vi "NI-DCPower Source DC Voltage T14.vi"() -> ()   [LabVIEW 2021, in "NI-DCPower Source DC Voltage T14.lvlib"]
doc: "Demonstrates how to use the DC Voltage Output Function to force an output voltage. This example initializes a session, configures the Output Function, Sense, Autorange, Voltage Level and Current Limit, initiates generation, waits for a specified delay, and measures the voltage and current output. This example uses Single Point source mode."
uses:
  NI-DCPower Source DC Voltage T14.lvlib
  <instrlib>/niDCPower/nidcpower.llb/niDCPower Source Mode.ctl
  <instrlib>/niDCPower/nidcpower.llb/niDCPower Wait For Event - Event.ctl
  <instrlib>/niDCPower/nidcpower.llb/niDCPower Output Function.ctl
panel:
  in  "error in":errorcluster
  out "error out":errorcluster
  in  "Source Delay (Sec)":dbl=0.1 format="%.3p"
  out "Voltage Measurement":dbl
  out "Current Measurement":dbl
  in  "Current Limit Range":dbl=0.01 format="%.3p"
  in  "Voltage Level Range":dbl=6.0 format="%.5p"
  in  "Current Limit":dbl=0.01 format="%.3p"
  in  "Voltage Level":dbl=2.0 format="%.5p"
  in  "Vin SMU Channel":string="0"
  in  "Vin SMU":refnum<k15>="Dev1"
  # "Overview: Demonstrates how to use the DC Voltage Output Function to force an output voltage.  \nThis example initializes a session; configures the Output Function, Voltage Level and Current Limit; \ninitiates generation; waits for a specified delay; and measures the voltage and current output. \nRequirements: NI-DCPower\nInstructions:\n1. Select the appropriate device in the Resource Name control.\n2. Configure the parameters of the DC Voltage signal you'd like to output.\n3. Run the VI."
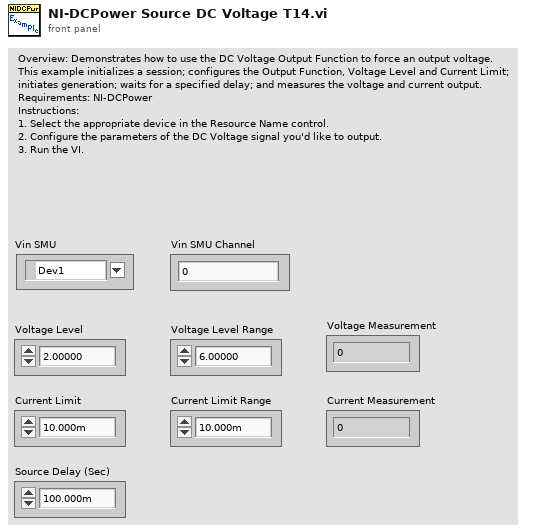
[diagram p1: front panel]
types:
  T1 = typedef "niDCPower Output Function.ctl" = i32
  T2 = typedef "niDCPower Wait For Event - Event.ctl" = i32
  T3 = typedef "niDCPower Source Mode.ctl" = i32
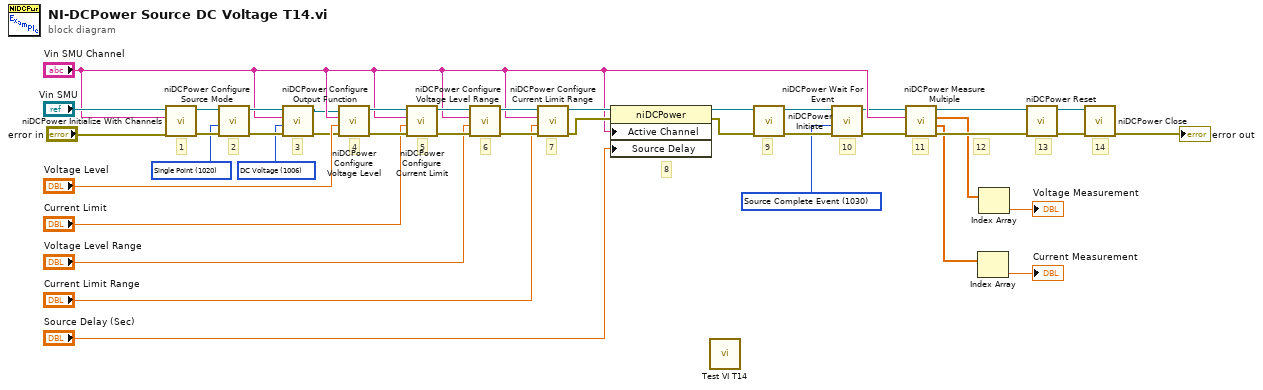
[diagram p0: block diagram]
diagram:
  w7 = T1 1006 items=["DC Voltage"=1006, "DC Current"=1007, "Pulse Voltage"=1049, "Pulse Current"=1050] ("output function")
  w10 = T2 1030 items=["Source Complete Event"=1030, "Measure Complete Event"=1031, "Sequence Iteration Complete Event"=1032, "Sequence Engine Done Event"=1033] ("event")
  w29 = T3 1020 items=["Single Point"=1020, "Sequence"=1021] ("source mode")
  # "14"
  # "9"
  # "11"
  # "10"
  # "7"
  # "6"
  # "2"
  # "3"
  # "12"
  # "13"
  # "8"
  # "5"
  # "4"
  # "1"
  n1 = call <instrlib>:"niDCPower Initialize With Channels.vi"("error in (no error)"="error in", "channels"="Vin SMU Channel", "resource name"="Vin SMU") -> ("error out"=w33:errorcluster, "instrument handle out"=w32:refnum<k15>)  [unwired: 2 in, 5 out]
  n2 = call <instrlib>:"niDCPower Configure Source Mode.vi"("error in (no error)"=w33, "source mode"=w29, "instrument handle"=w32) -> ("error out"=w31:errorcluster, "instrument handle out"=w30:refnum<k15>)  [unwired: 7 out]
  n3 = call <instrlib>:"niDCPower Configure Output Function.vi"("error in (no error)"=w31, "output function"=w7, "channel name"="Vin SMU Channel", "instrument handle"=w30) -> ("error out"=w8:errorcluster, "instrument handle out"=w9:refnum<k15>)  [unwired: 6 out]
  n4 = call <instrlib>:"niDCPower Configure Voltage Level.vi"("error in (no error)"=w8, "voltage level"="Voltage Level", "channel name"="Vin SMU Channel", "instrument handle"=w9) -> ("error out"=w38:errorcluster, "instrument handle out"=w39:refnum<k15>)  [unwired: 6 out]
  n5 = call <instrlib>:"niDCPower Configure Current Limit.vi"("error in (no error)"=w38, "current limit"="Current Limit", "channel name"="Vin SMU Channel", "instrument handle"=w39) -> ("error out"=w28:errorcluster, "instrument handle out"=w27:refnum<k15>)  [unwired: 1 in, 5 out]
  n6 = call <instrlib>:"niDCPower Configure Voltage Level Range.vi"("error in (no error)"=w28, "voltage level range"="Voltage Level Range", "channel name"="Vin SMU Channel", "instrument handle"=w27) -> ("error out"=w26:errorcluster, "instrument handle out"=w25:refnum<k15>)  [unwired: 6 out]
  n7 = call <instrlib>:"niDCPower Configure Current Limit Range.vi"("error in (no error)"=w26, "current limit range"="Current Limit Range", "channel name"="Vin SMU Channel", "instrument handle"=w25) -> ("error out"=w17:errorcluster, "instrument handle out"=w20:refnum<k15>)  [unwired: 6 out]
  n8 = property class="niDCPower"(reference=w20, error in=w17, "Active Channel"="Vin SMU Channel", "Source Delay"="Source Delay (Sec)") -> (reference out=w19:refnum<k15>, error out=w18:errorcluster)
  n9 = call "Test VI T14.vi"() -> ()  [unwired: 16 in]
  n10 = call <instrlib>:"niDCPower Initiate.vi"("error in (no error)"=w18, "instrument handle"=w19) -> ("error out"=w12:errorcluster, "instrument handle out"=w14:refnum<k15>)  [unwired: 2 in, 6 out]
  n11 = call <instrlib>:"niDCPower Wait For Event.vi"("error in (no error)"=w12, "event"=w10, "instrument handle"=w14) -> ("error out"=w11:errorcluster, "instrument handle out"=w13:refnum<k15>)  [unwired: 1 in, 6 out]
  n12 = call <instrlib>:"niDCPower Measure Multiple.vi"("error in (no error)"=w11, "channel name"="Vin SMU Channel", "instrument handle"=w13) -> ("error out"=w21:errorcluster, "current measurements"=w4:dbl[], "voltage measurements"=w2:dbl[], "instrument handle out"=w22:refnum<k15>)  [unwired: 5 out]
  n13 = Index Array(array=w4) -> (element=→"Current Measurement":dbl)  [unwired: 1 in]
  n14 = Index Array(array=w2) -> (element=→"Voltage Measurement":dbl)  [unwired: 1 in]
  n15 = call <instrlib>:"niDCPower Reset.vi"("error in (no error)"=w21, "instrument handle"=w22) -> ("error out"=w35:errorcluster, "instrument handle out"=w36:refnum<k15>)  [unwired: 2 in, 6 out]
  n16 = call <instrlib>:"niDCPower Close.vi"("error in (no error)"=w35, "instrument handle"=w36) -> ("error out"=→"error out":errorcluster)  [unwired: 9 out]
